vi "Write Data Attributes.vi"(8 "error in (no error)":errorcluster, 10 "data attributes":variant, 11 "Data in":refnum<class "Data.lvclass">) -> (0 "error out":errorcluster, 3 "Data out":refnum<class "Data.lvclass">)   [LabVIEW 2017, in "Data.lvclass"]
uses:
  <vilib>/addons/_NISVFA/_Shared subVIs/Data Objects/Data/Data.lvclass
  <vilib>/addons/_NISVFA/_Shared subVIs/Data Objects/Data/Data.lvclass/Data.ctl
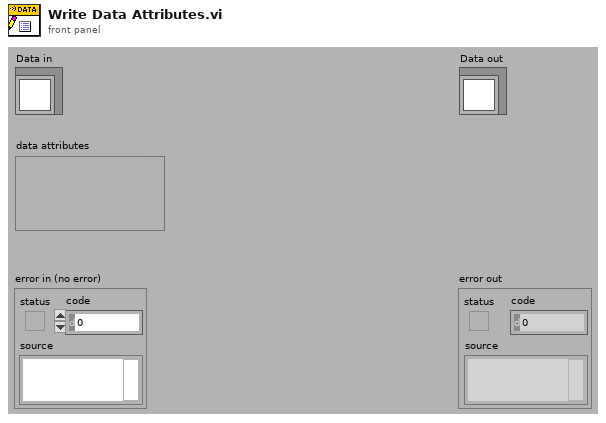
[diagram p1: front panel]
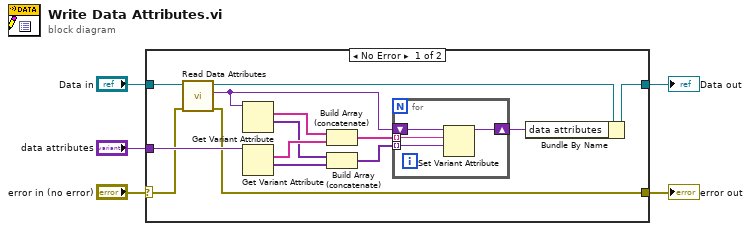
[diagram p0: block diagram]
diagram:
  n1 = case shown="No Error" "error in (no error)" {
    selector: "error in (no error)" -> [w7 w24]
    tunnel: [w6 w24] -> w4
    tunnel: [w19 w25] -> w2
    tunnel: "Data in" -> [w18 w25]
    tunnel: "data attributes" -> [w17 _]
    frame No Error {
      n2 = call <vilib>:"Read Data Attributes.vi"("error in (no error)"=w7, "Data in"=w18) -> ("error out"=w6:errorcluster, "data attributes"=w12:variant, "Data out"=w8:refnum<class "Data.lvclass">)  [unwired: 7 in]
      n3 = Get Variant Attribute(Variant=w12) -> (names=w16:string[], values=w13:variant[])  [unwired: 3 in, 2 out]
      n4 = Get Variant Attribute(Variant=w17) -> (names=w15:string[], values=w14:variant[])  [unwired: 3 in, 2 out]
      n5 = Build Array (concatenate)(w16, w15) -> (w11:string[])
      n6 = Build Array (concatenate)(w13, w14) -> (w10:variant[])
      n7 = for {
        shift-right: [w22] -> w9
        shift-left: w12 -> [w23]
        tunnel: w11 -> [w21] mode=indexing
        tunnel: w10 -> [w20] mode=indexing
        n8 = Set Variant Attribute(Variant=w23, name=w21, value=w20) -> (Variant out=w22:variant)  [unwired: 1 in, 2 out]
      }
      n9 = Bundle By Name(cluster=w8, "data attributes"=w9) -> (w19:refnum<class "Data.lvclass">)
    }
    frame Error {
    }
  }
  "error out" <- w4
  "Data out" <- w2
